vi "Begin.vi"(8 "error in":errorcluster) -> (0 "error out":errorcluster)   [LabVIEW 2020]
doc: "Called before other user functions, this VI is expected to open initial I/O refnums, load in file data, and do all program initialization. Notice that the <B>error out</B> terminal is simply used for data flow. Wiring it to other structures or subVIs ensures that this VI runs first."
uses:
  <vilib>/Rock Robotics/WPI/Joystick/WPI_JoystickDeviceEnum.ctl
  Shared Code/TypeDefs/ENUM_AutoSelect.ctl
  e0c29a47-0ff2-46a8-a53f-5c1cdae12b99.vi
  Utility/Global_STOP.vi
  Robot Global Data.vi
  Systems/SwerveOdometry/Global_CMD_SEN_Data In.vi
  Systems/SwerveOdometry/Swerve_Odometry_SEN.lvlib
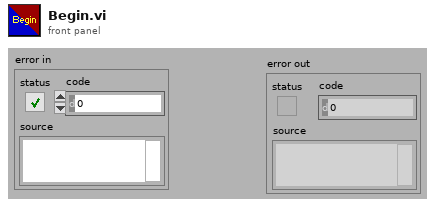
[diagram p1: front panel]
types:
  T1 = typedef "ENUM_AutoSelect.ctl" = enum16{"Unknown", "Drop Mid Drive Straight", "Drop mid dock and engage", "Drop High dock and engage", "Drop Low dock and engage", "Manual", "Over and Rebalance", "Over and Dock"}
  T2 = typedef "WPI_JoystickDeviceEnum.ctl" = enum16{"USB 0", "USB 1", "USB 2", "USB 3", "USB 4", "USB 5"}
  T3 = typedef "WPI_Joystick Info.ctl" = cluster{"Device Name":string, "HID Type":T4, "XBox Type":T5, "Axes Count":i32, "Axes Types":T6[], "Button Count":i32, "POV Count":i32}
  T4 = typedef "WPI_JoystickHID Types.ctl" = enum16{"Not HID", "HID Joystick", "HID Gamepad", "HID Driving Wheel", "HID Flightstick", "HID First Person"}
  T5 = typedef "WPI_JoystickXBox Types.ctl" = enum16{"Not XBox", "XBox Unknown", "XBox Gamepad", "XBox Wheel", "XBox Arcade Stick", "XBox Flight Stick", "XBox Dance Pad", "XBox Guitar", "XBox Drum Kit", "XBox Arcade Pad"}
  T6 = typedef "WPI_JoystickAxis Types.ctl" = enum16{"X Axis", "Y Axis", "Z Axis", "RxAxis", "RyAxis", "RzAxis", "Slider", "POV", "None", "L X Axis", "L Y Axis", "L Trigger", "R Trigger", "R X Axis", "R Y Axis"}
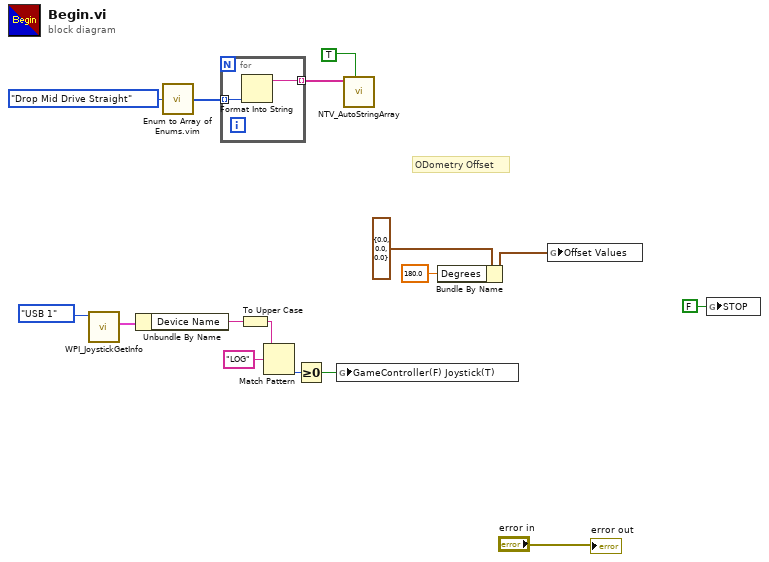
[diagram p0: block diagram]
diagram:
  # "ODometry Offset"
  n1 = call <vilib>:"WPI_JoystickGetInfo.vi"("JoystickDevice"=WPI_JoystickDeviceEnum."USB 1") -> ("Joystick Info"=w14:T3)  [unwired: 9 in, 1 out]
  n2 = Unbundle By Name(w14) -> ("Device Name"=w13:string)
  n3 = call "Enum to Array of Enums.vim"("enum"=ENUM_AutoSelect."Drop Mid Drive Straight" ("Auto Select")) -> ("array of enums"=w5:T1[])
  n4 = for {
    tunnel: w5 -> [w18] mode=indexing
    tunnel: [w17] -> w4 mode=indexing
    n5 = Format Into String(w18) -> (resulting string=w17:string)  [unwired: 3 in, 1 out]
  }
  n6 = To Upper Case(1:w13) -> (0:w11:string)
  n7 = Match Pattern(string=w11, regular expression="LOG") -> (offset past match=w10:i32)  [unwired: 1 in, 3 out]
  n8 = Greater Or Equal To 0?(x=w10) -> (x >= 0?=w9:bool)
  n9 = global write "Robot Global Data.vi" "GameController(F) Joystick(T)"(w9) -> ()
  n10 = call "NTV_AutoStringArray.vi"("Read(f) Write(t)"=TRUE, "Array"=w4) -> ()  [unwired: 9 in, 1 out]
  n11 = Bundle By Name(cluster=cluster{"Y":dbl, "X":dbl, "Degrees":dbl} {"Y"=0.0, "X"=0.0, "Degrees"=0.0} ("Offset Values"), "Degrees"=180.0) -> (w2:cluster{"Y":dbl, "X":dbl, "Degrees":dbl})
  n12 = global write "Global_CMD_SEN_Data In.vi" "Offset Values"(w2) -> ()
  n13 = global write "Global_STOP.vi" "STOP"(FALSE ("STOP")) -> ()
  "error out" <- "error in"
